vi "ma_Spectrum compensation from other tones.vi"(1 "other tones' information":T3(array[cluster]) {"phase [degree]" format="%.2f"; "amplitude" format="%.2f"; "frequency" format="%.2f"}, 2 "spectral info":T2 {"window" items=["Rectangle"=0, "Hanning"=1, "Hamming"=2, "Blackman-Harris"=3, "Exact Blackman"=4, "Blackman"=5, "Flat Top"=6, "4 Term B-Harris "=7, "7 Term B-Harris"=8, "Low Sidelobe"=9, "Blackman Nuttall"=11, "Triangle"=30, "Bartlett-Hanning"=31, "Bohman"=32, "Parzen"=33, "Welch"=34, "Kaiser"=60, "Dolph-Chebyshev"=61, "Gaussian"=62]}, 3 "FFT spectrum":T1={"f0"=0.0, "df"=1.0, "spectrum"=[]} {"spectrum" format="%.2f"; "df" format="%.2f"; "f0" format="%.2f"}) -> (0 "compensated FFT spectrum":T1={"f0"=0.0, "df"=1.0, "spectrum"=[]} {"spectrum" format="%.2f"; "df" format="%.2f"; "f0" format="%.2f"})   [LabVIEW 2020, in "NI_MAPro.lvlib"]
uses:
  NI_MAPro.lvlib
  ma_sml_Spectral Info.ctl
  ma_sml_Spectrum Cluster (complex).ctl
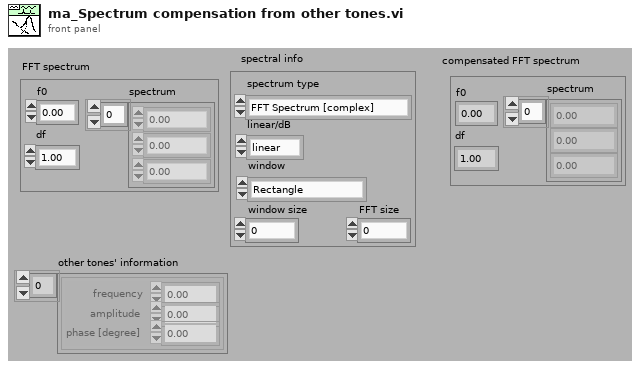
[diagram p1: front panel]
types:
  T1 = typedef "NI_MAPro.lvlib/ma_sml_Spectrum Cluster (complex).ctl" = cluster{"f0":dbl, "df":dbl, "spectrum":cdb[]}
  T2 = typedef "NI_MAPro.lvlib/ma_sml_Spectral Info.ctl" = cluster{"spectrum type":enum16{"FFT Spectrum [complex]", "Amplitude [Magnitude]", "Power [Magnitude^2]", "Cross Spectrum [complex]", "Frequency Response [Complex]"}, "linear/dB":enum16{"linear", "dB"}, "window":u16, "window size":i32, "FFT size":i32}
  T3 = cluster{"frequency":dbl, "amplitude":dbl, "phase [degree]":dbl}[]
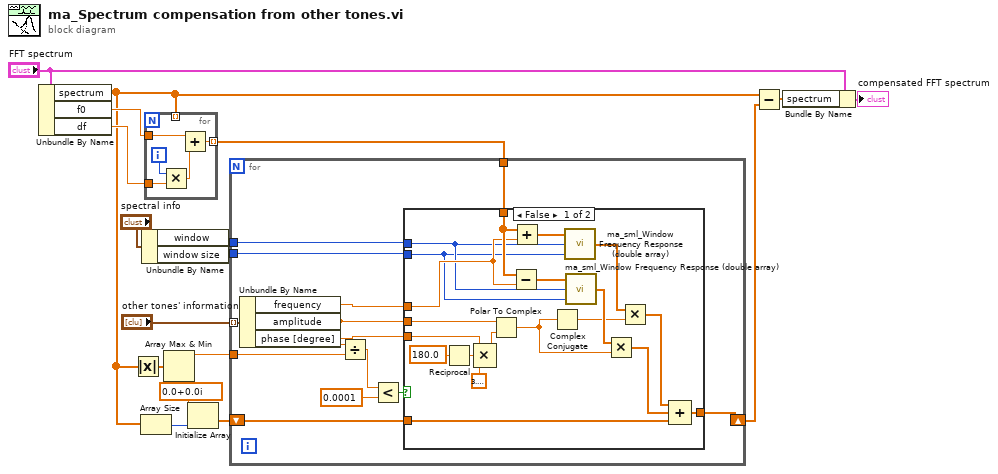
[diagram p0: block diagram]
diagram:
  n1 = Unbundle By Name("FFT spectrum") -> ("spectrum"=w3:cdb[], "f0"=w8:dbl, "df"=w7:dbl)
  n2 = Absolute Value(x=w3) -> (abs(x)=w2:dbl[])
  n3 = Array Size(array=w3) -> (size(s)=w4:i32)
  n4 = Unbundle By Name("spectral info") -> ("window"=w6:u16, "window size"=w5:i32)
  n5 = for {
    tunnel: w8 -> [w22]
    tunnel: w7 -> [w20]
    tunnel: [w18] -> w16 mode=indexing
    tunnel: w3 -> [_] mode=indexing
    i -> [w21]
    n6 = Multiply(x=w21, y=w20) -> (x*y=w19:dbl)
    n7 = Add(x=w22, y=w19) -> (x+y=w18:dbl)
  }
  n8 = Array Max & Min(array=w2) -> (max value=w1:dbl)  [unwired: 3 out]
  n9 = Initialize Array(cdb 0.0+0.0i ("Element Data"), w4) -> (w10:cdb[])
  n10 = for {
    tunnel: "other tones' information" -> [w35] mode=indexing
    tunnel: w16 -> [w31]
    shift-right: [w32] -> w15
    shift-left: w10 -> [w33]
    tunnel: w6 -> [w28]
    tunnel: w5 -> [w27]
    tunnel: w1 -> [w26]
    n11 = Unbundle By Name(w35) -> ("frequency"=w30:dbl, "amplitude"=w25:dbl, "phase [degree]"=w34:dbl)
    n12 = Divide(x=w25, y=w26) -> (x/y=w24:dbl)
    n13 = Less?(x=w24, y=0.0001) -> (x < y?=w29:bool)
    n14 = case shown="False" w29 {
      tunnel: w34 -> [w55 _]
      tunnel: w25 -> [w52 _]
      tunnel: w30 -> [w38 _]
      tunnel: w33 -> [w46 w56]
      tunnel: [w45 w56] -> w32
      tunnel: w31 -> [w40 _]
      tunnel: w28 -> [w37 _]
      tunnel: w27 -> [w36 _]
      frame False {
        n15 = Reciprocal(x=180.0 ("y")) -> (1/x=w39:dbl)
        n16 = Compound Arithmetic op=MULTIPLY(w55, w39, 3.141592653589793) -> (w51:dbl)
        n17 = Polar To Complex(1:w51, 2:w52) -> (0:w43:cdb)
        n18 = Subtract(x=w40, y=w38) -> (x-y=w49:dbl[])
        n19 = Add(x=w40, y=w38) -> (x+y=w50:dbl[])
        n20 = Complex Conjugate(1:w43) -> (0:w42:cdb)
        n21 = call "ma_sml_Window Frequency Response (double array).vi"("N (window length)"=w36, "window"=w37, "f(normalized)"=w50) -> ("H(f)"=w48:cdb[])
        n22 = call "ma_sml_Window Frequency Response (double array).vi"("N (window length)"=w36, "window"=w37, "f(normalized)"=w49) -> ("H(f)"=w47:cdb[])
        n23 = Multiply(x=w47, y=w43) -> (x*y=w41:cdb[])
        n24 = Multiply(x=w48, y=w42) -> (x*y=w44:cdb[])
        n25 = Compound Arithmetic op=ADD(w44, w41, w46) -> (w45:cdb[])
      }
      frame True {
      }
    }
  }
  n26 = Subtract(x=w3, y=w15) -> (x-y=w12:cdb[])
  n27 = Bundle By Name(cluster="FFT spectrum", "spectrum"=w12) -> (→"compensated FFT spectrum":T1)
